vi "ReadSSF_DSF.vi"(10 "DRWM path 2":path, 11 "DRWM path 1":path) -> (0 "DSF":cluster{"x":dbl, "y":dbl}[][](array[cluster]), 1 "因子棒号":string[](array[string]), 2 "SF_0K":bool, 3 "SSF":cluster{"x":dbl, "y":dbl}[][](array[cluster]), 5 "文件INFO":string)   [LabVIEW 2020]
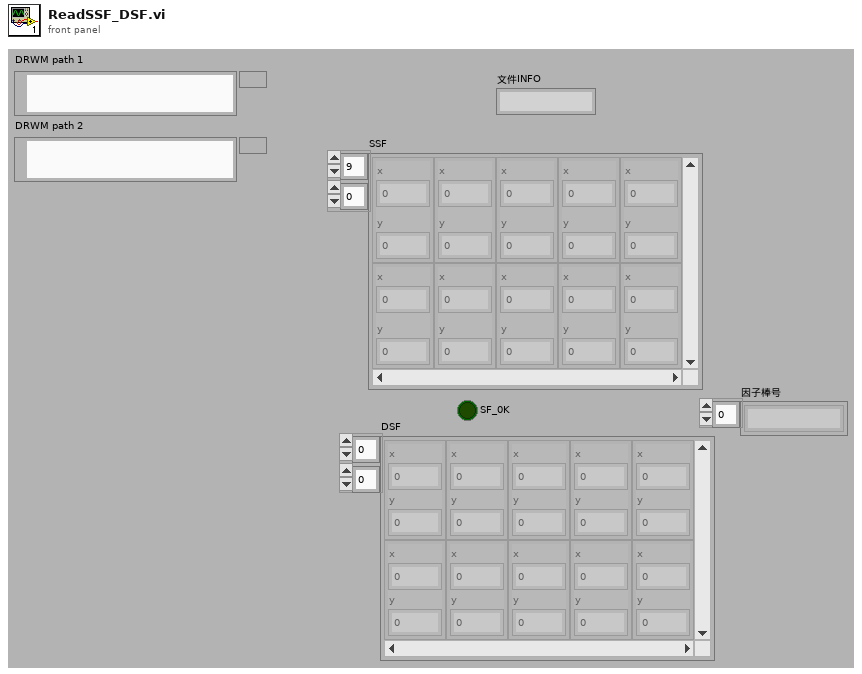
[diagram p1: front panel]
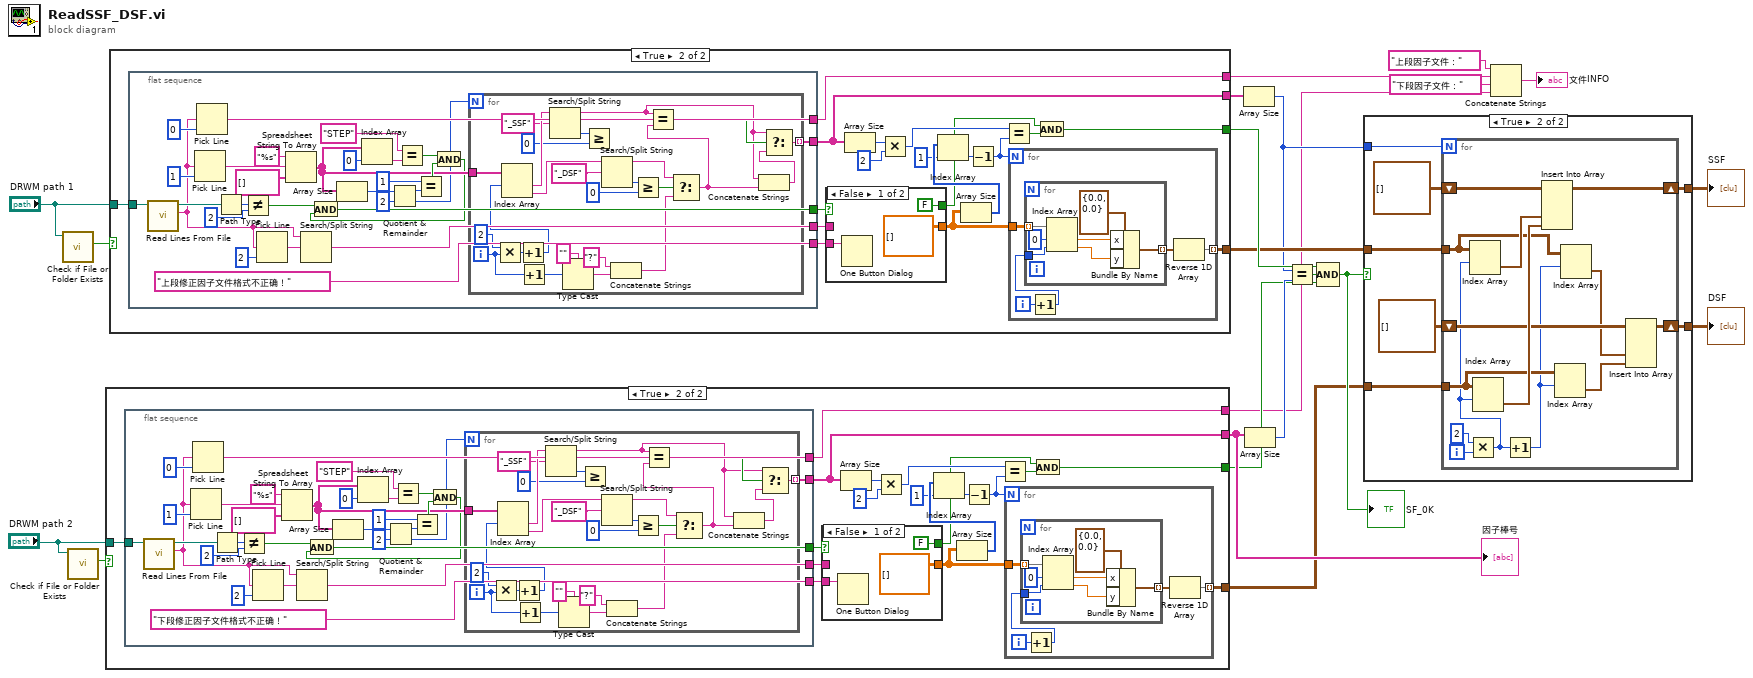
[diagram p0: block diagram]
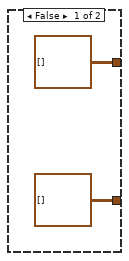
[diagram p2: hidden frame]
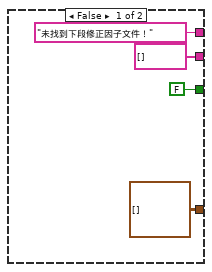
[diagram p3: hidden frame]
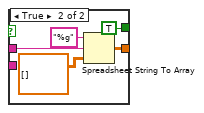
[diagram p4: hidden frame]
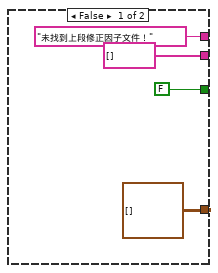
[diagram p5: hidden frame]
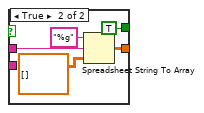
[diagram p6: hidden frame]
diagram:
  n1 = call <vilib>:"Check if File or Folder Exists.vi"("path"="DRWM path 1") -> ("file or folder exists?"=w21:bool)  [unwired: 8 in, 2 out]
  n2 = call <vilib>:"Check if File or Folder Exists.vi"("path"="DRWM path 2") -> ("file or folder exists?"=w20:bool)  [unwired: 8 in, 2 out]
  n3 = case shown="True" w20 {
    tunnel: [cluster{"x":dbl, "y":dbl}[][] [] w39] -> w12
    tunnel: "DRWM path 2" -> [_ w40]
    tunnel: [FALSE ("file or folder exists?") w28] -> w15
    tunnel: ["未找到下段修正因子文件！" ("output string") w27] -> w3
    tunnel: [string[] [] w26] -> w18
    frame False {
    }
    frame True {
      n4 = flat-sequence {
        tunnel: [w81] -> w43
        tunnel: [w73] -> w42
        tunnel: ["下段修正因子文件格式不正确！" ("消息")] -> w41
        tunnel: w40 -> [w78]
        tunnel: [w72] -> w27
        tunnel: [w57] -> w26
        frame #0 {
          n5 = call <vilib>:"Read Lines From File.vi"("file path (dialog if empty)"=w78) -> ("new file path (Not A Path if cancelled)"=w80:path, "line string"=w74:string)  [unwired: 5 in, 2 out]
          n6 = Pick Line ("选行并添加至字符串")(multi-line string=w74, line index=1 ("行索引")) -> (output string=w70:string)  [unwired: 1 in]
          n7 = Pick Line ("选行并添加至字符串")(multi-line string=w74, line index=0 ("行索引")) -> (output string=w72:string)  [unwired: 1 in]
          n8 = Path Type(1:w80) -> (0:w84:i16)
          n9 = Not Equal?(x=w84, y=i16 2) -> (x != y?=w82:bool)
          n10 = Pick Line ("选行并添加至字符串")(multi-line string=w74, line index=2 ("行索引")) -> (output string=w75:string)  [unwired: 1 in]
          n11 = Spreadsheet String To Array ("电子表格字符串至数组转换")(format string="%s" ("format (%.3f)"), spreadsheet string=w70, array type (2D Dbl)=string[] [] ("添加的数组")) -> (array=w59:string[])  [unwired: 1 in]
          n12 = Search/Split String(string=w74, search string/char (-)=w75) -> (match + rest of string=w73:string)  [unwired: 1 in, 2 out]
          n13 = Array Size(array=w59) -> (size(s)=w65:i32)
          n14 = Index Array(array=w59, index=0 ("索引")) -> (element=w67:string)
          n15 = Quotient & Remainder(x=w65, y=2) -> (x-y*floor(x/y)=w63:i32, floor(x/y)=w58:i32)
          n16 = Equal?(x="STEP", y=w67) -> (x = y?=w60:bool)
          n17 = Equal?(x=1, y=w63) -> (x = y?=w61:bool)
          n18 = And(x=w60, y=w61) -> (x .and. y?=w56:bool)
          n19 = And(x=w82, y=w56) -> (x .and. y?=w81:bool)
          n20 = for {
            N: w58 -> [_]
            tunnel: w59 -> [w110]
            tunnel: [w94] -> w57 mode=indexing
            i -> [w96]
            n21 = Multiply(x=2, y=w96) -> (x*y=w108:i32)
            n22 = Increment(x=w108) -> (x+1=w107:i32)
            n23 = Index Array(array=w110, index #1=w107) -> (element #1=w106:string, element #2=w99:string)  [unwired: 1 in]
            n24 = Increment(x=w96) -> (x+1=w95:i32)
            n25 = Search/Split String(string=w106, search string/char (-)="_SSF" ("搜索字符串/字符(-)")) -> (substring before match=w89:string, offset of match=w104:i32)  [unwired: 1 in, 1 out]
            n26 = Type Cast(type="" ("类型"), x=w95) -> (*(type *) &x=w93:string)
            n27 = Greater Or Equal?(x=w104, y=0) -> ()  [unwired: 1 out]
            n28 = Search/Split String(string=w99, search string/char (-)="_DSF" ("搜索字符串/字符(-)")) -> (substring before match=w91:string, offset of match=w101:i32)  [unwired: 1 in, 1 out]
            n29 = Concatenate Strings("?" ("字符串"), w93) -> (w88:string)
            n30 = Greater Or Equal?(x=w101, y=0) -> (x >= y?=w86:bool)
            n31 = Select(t=w91, s=w86, f=w88) -> (s? t:f=w87:string)
            n32 = Equal?(x=w89, y=w87) -> (x = y?=w98:bool)
            n33 = Concatenate Strings(w89, w87) -> (w90:string)
            n34 = Select(t=w89, s=w98, f=w90) -> (s? t:f=w94:string)
          }
        }
      }
      n35 = case shown="False" w43 {
        tunnel: w42 -> [_ w115]
        tunnel: [dbl[][] [] ("type (empty)") w116] -> w38
        tunnel: w41 -> [w112 _]
        tunnel: [FALSE ("file or folder exists?") TRUE ("file or folder exists?")] -> w29
        frame False {
          n36 = One Button Dialog(message=w112) -> ()  [unwired: 1 in, 1 out]
        }
        frame True {
          n37 = Spreadsheet String To Array ("电子表格字符串至数组转换")(format string="%g" ("format (%.3f)"), spreadsheet string=w115, array type (2D Dbl)=dbl[][] [] ("type (empty)")) -> (array=w116:dbl[][])  [unwired: 1 in]
        }
      }
      n38 = Array Size(array=w26) -> (size(s)=w34:i32)
      n39 = Multiply(x=w34, y=2) -> (x*y=w32:i32)
      n40 = Array Size(array=w38) -> (size(s)=w37:i32[])
      n41 = Index Array(array=w37, index=1 ("索引")) -> (element=w35:i32)
      n42 = Decrement(x=w35) -> (x-1=w31:i32)
      n43 = Equal?(x=w32, y=w31) -> (x = y?=w30:bool)
      n44 = for {
        N: w31 -> [_]
        tunnel: w38 -> [w47]
        tunnel: [w46] -> w39 mode=indexing
        i -> [w44]
        n45 = Increment(x=w44) -> (x+1=w45:i32)
        n46 = for {
          tunnel: w47 -> [w55] mode=indexing
          tunnel: [w53] -> w48 mode=indexing
          tunnel: w45 -> [w49]
          n47 = Index Array(array=w55, index #1=0 ("索引"), index #2=w49) -> (element #1=w51:dbl, element #2=w54:dbl)
          n48 = Bundle By Name(cluster=cluster{"x":dbl, "y":dbl} {"x"=0.0, "y"=0.0} ("输入簇"), "x"=w51, "y"=w54) -> (w53:cluster{"x":dbl, "y":dbl})
        }
        n49 = Reverse 1D Array(array=w48) -> (reversed array=w46:cluster{"x":dbl, "y":dbl}[])
      }
      n50 = And(x=w29, y=w30) -> (x .and. y?=w28:bool)
    }
  }
  "因子棒号" <- w18
  n51 = case shown="True" w21 {
    tunnel: [cluster{"x":dbl, "y":dbl}[][] [] w136] -> w13
    tunnel: "DRWM path 1" -> [_ w137]
    tunnel: [FALSE ("file or folder exists?") w125] -> w16
    tunnel: ["未找到上段修正因子文件！" ("output string") w124] -> w6
    tunnel: [string[] [] w123] -> w19
    frame False {
    }
    frame True {
      n52 = flat-sequence {
        tunnel: [w178] -> w140
        tunnel: [w170] -> w139
        tunnel: ["上段修正因子文件格式不正确！" ("消息")] -> w138
        tunnel: w137 -> [w175]
        tunnel: [w169] -> w124
        tunnel: [w154] -> w123
        frame #0 {
          n53 = call <vilib>:"Read Lines From File.vi"("file path (dialog if empty)"=w175) -> ("new file path (Not A Path if cancelled)"=w177:path, "line string"=w171:string)  [unwired: 5 in, 2 out]
          n54 = Pick Line ("选行并添加至字符串")(multi-line string=w171, line index=1 ("行索引")) -> (output string=w167:string)  [unwired: 1 in]
          n55 = Pick Line ("选行并添加至字符串")(multi-line string=w171, line index=0 ("行索引")) -> (output string=w169:string)  [unwired: 1 in]
          n56 = Path Type(1:w177) -> (0:w181:i16)
          n57 = Not Equal?(x=w181, y=i16 2) -> (x != y?=w179:bool)
          n58 = Pick Line ("选行并添加至字符串")(multi-line string=w171, line index=2 ("行索引")) -> (output string=w172:string)  [unwired: 1 in]
          n59 = Spreadsheet String To Array ("电子表格字符串至数组转换")(format string="%s" ("format (%.3f)"), spreadsheet string=w167, array type (2D Dbl)=string[] [] ("添加的数组")) -> (array=w156:string[])  [unwired: 1 in]
          n60 = Search/Split String(string=w171, search string/char (-)=w172) -> (match + rest of string=w170:string)  [unwired: 1 in, 2 out]
          n61 = Array Size(array=w156) -> (size(s)=w162:i32)
          n62 = Index Array(array=w156, index=0 ("索引")) -> (element=w164:string)
          n63 = Quotient & Remainder(x=w162, y=2) -> (x-y*floor(x/y)=w160:i32, floor(x/y)=w155:i32)
          n64 = Equal?(x="STEP", y=w164) -> (x = y?=w157:bool)
          n65 = Equal?(x=1, y=w160) -> (x = y?=w158:bool)
          n66 = And(x=w157, y=w158) -> (x .and. y?=w153:bool)
          n67 = And(x=w179, y=w153) -> (x .and. y?=w178:bool)
          n68 = for {
            N: w155 -> [_]
            tunnel: w156 -> [w207]
            tunnel: [w191] -> w154 mode=indexing
            i -> [w193]
            n69 = Multiply(x=2, y=w193) -> (x*y=w205:i32)
            n70 = Increment(x=w205) -> (x+1=w204:i32)
            n71 = Index Array(array=w207, index #1=w204) -> (element #1=w203:string, element #2=w196:string)  [unwired: 1 in]
            n72 = Increment(x=w193) -> (x+1=w192:i32)
            n73 = Search/Split String(string=w203, search string/char (-)="_SSF" ("搜索字符串/字符(-)")) -> (substring before match=w186:string, offset of match=w201:i32)  [unwired: 1 in, 1 out]
            n74 = Type Cast(type="" ("类型"), x=w192) -> (*(type *) &x=w190:string)
            n75 = Greater Or Equal?(x=w201, y=0) -> ()  [unwired: 1 out]
            n76 = Search/Split String(string=w196, search string/char (-)="_DSF" ("搜索字符串/字符(-)")) -> (substring before match=w188:string, offset of match=w198:i32)  [unwired: 1 in, 1 out]
            n77 = Concatenate Strings("?" ("字符串"), w190) -> (w185:string)
            n78 = Greater Or Equal?(x=w198, y=0) -> (x >= y?=w183:bool)
            n79 = Select(t=w188, s=w183, f=w185) -> (s? t:f=w184:string)
            n80 = Equal?(x=w186, y=w184) -> (x = y?=w195:bool)
            n81 = Concatenate Strings(w186, w184) -> (w187:string)
            n82 = Select(t=w186, s=w195, f=w187) -> (s? t:f=w191:string)
          }
        }
      }
      n83 = case shown="False" w140 {
        tunnel: w139 -> [_ w212]
        tunnel: [dbl[][] [] ("type (empty)") w213] -> w135
        tunnel: w138 -> [w209 _]
        tunnel: [FALSE ("file or folder exists?") TRUE ("file or folder exists?")] -> w126
        frame False {
          n84 = One Button Dialog(message=w209) -> ()  [unwired: 1 in, 1 out]
        }
        frame True {
          n85 = Spreadsheet String To Array ("电子表格字符串至数组转换")(format string="%g" ("format (%.3f)"), spreadsheet string=w212, array type (2D Dbl)=dbl[][] [] ("type (empty)")) -> (array=w213:dbl[][])  [unwired: 1 in]
        }
      }
      n86 = Array Size(array=w123) -> (size(s)=w131:i32)
      n87 = Multiply(x=w131, y=2) -> (x*y=w129:i32)
      n88 = Array Size(array=w135) -> (size(s)=w134:i32[])
      n89 = Index Array(array=w134, index=1 ("索引")) -> (element=w132:i32)
      n90 = Decrement(x=w132) -> (x-1=w128:i32)
      n91 = Equal?(x=w129, y=w128) -> (x = y?=w127:bool)
      n92 = for {
        N: w128 -> [_]
        tunnel: w135 -> [w144]
        tunnel: [w143] -> w136 mode=indexing
        i -> [w141]
        n93 = Increment(x=w141) -> (x+1=w142:i32)
        n94 = for {
          tunnel: w144 -> [w152] mode=indexing
          tunnel: [w150] -> w145 mode=indexing
          tunnel: w142 -> [w146]
          n95 = Index Array(array=w152, index #1=0 ("索引"), index #2=w146) -> (element #1=w148:dbl, element #2=w151:dbl)
          n96 = Bundle By Name(cluster=cluster{"x":dbl, "y":dbl} {"x"=0.0, "y"=0.0} ("输入簇"), "x"=w148, "y"=w151) -> (w150:cluster{"x":dbl, "y":dbl})
        }
        n97 = Reverse 1D Array(array=w145) -> (reversed array=w143:cluster{"x":dbl, "y":dbl}[])
      }
      n98 = And(x=w126, y=w127) -> (x .and. y?=w125:bool)
    }
  }
  n99 = Array Size(array=w19) -> (size(s)=w11:i32)
  n100 = Array Size(array=w18) -> (size(s)=w17:i32)
  n101 = Equal?(x=w11, y=w17) -> (x = y?=w10:bool)
  n102 = Compound Arithmetic op=AND(w16, w10, w15) -> (w14:bool)
  "SF_0K" <- w14
  n103 = case shown="True" w14 {
    tunnel: w13 -> [_ w223]
    tunnel: w12 -> [_ w222]
    tunnel: w11 -> [_ w224]
    tunnel: [cluster{"x":dbl, "y":dbl}[][] [] w220] -> w9
    tunnel: [cluster{"x":dbl, "y":dbl}[][] [] w218] -> w8
    frame False {
    }
    frame True {
      n104 = for {
        N: w224 -> [_]
        tunnel: w223 -> [w230]
        tunnel: w222 -> [w229]
        shift-right: [w235] -> w220
        shift-left: cluster{"x":dbl, "y":dbl}[][] [] -> [w236]
        shift-right: [w231] -> w218
        shift-left: cluster{"x":dbl, "y":dbl}[][] [] -> [w232]
        i -> [w238]
        n105 = Multiply(x=2, y=w238) -> (x*y=w228:i32)
        n106 = Index Array(array=w230, index (row)=w228) -> (element=w234:cluster{"x":dbl, "y":dbl}[])  [unwired: 1 in]
        n107 = Index Array(array=w229, index (row)=w228) -> (element=w233:cluster{"x":dbl, "y":dbl}[])  [unwired: 1 in]
        n108 = Increment(x=w228) -> (x+1=w227:i32)
        n109 = Insert Into Array(array=w236, new element #1=w234, new element #2=w233) -> (w235:cluster{"x":dbl, "y":dbl}[][])  [unwired: 2 in]
        n110 = Index Array(array=w229, index (row)=w227) -> (element=w225:cluster{"x":dbl, "y":dbl}[])  [unwired: 1 in]
        n111 = Index Array(array=w230, index (row)=w227) -> (element=w226:cluster{"x":dbl, "y":dbl}[])  [unwired: 1 in]
        n112 = Insert Into Array(array=w232, new element #1=w226, new element #2=w225) -> (w231:cluster{"x":dbl, "y":dbl}[][])  [unwired: 2 in]
      }
    }
  }
  "SSF" <- w9
  "DSF" <- w8
  n113 = Concatenate Strings("上段因子文件：" ("字符串"), w6, "下段因子文件：" ("字符串"), w3) -> (→"文件INFO":string)
